vi "configure.vi"(8 "error in (no error)":errorcluster, 11 "PackedLibrary in":refnum<class "PackedLibrary.lvclass">) -> (0 "error out":errorcluster, 3 "PackedLibrary out":refnum<class "PackedLibrary.lvclass">)   [LabVIEW 2024, in "PackedLibrary.lvclass"]
uses:
  PackedLibrary.lvclass
  PackedLibrary.lvclass/PackedLibrary.ctl
  <vilib>/AppBuilder/AB_API/PPL/NI_AB_API_PPL.lvclass
  parent/Builder.lvclass
  D:/_repos/sandbox/github_p/labview-tools/cicd_tools/src/builders/parent/Builder.lvclass
  D:/_repos/sandbox/github_p/labview-tools/cicd_tools/src/builders/packed_library/PackedLibrary.lvclass
  C:/Program Files/National Instruments/LabVIEW 2024/vi.lib/AppBuilder/AB_API/Targetfile/NI_AB_API_Targetfile.lvclass
  C:/Program Files/National Instruments/LabVIEW 2024/vi.lib/AppBuilder/AB_API/Build/NI_AB_API_Build.lvclass
  C:/Program Files/National Instruments/LabVIEW 2024/vi.lib/AppBuilder/AB_API/PPL/NI_AB_API_PPL.lvclass
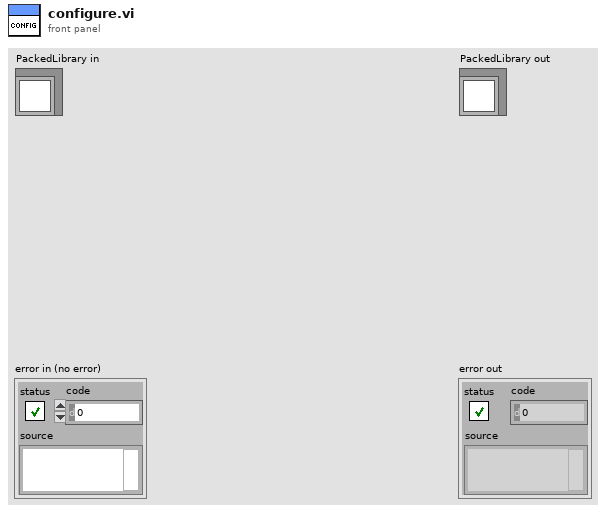
[diagram p1: front panel]
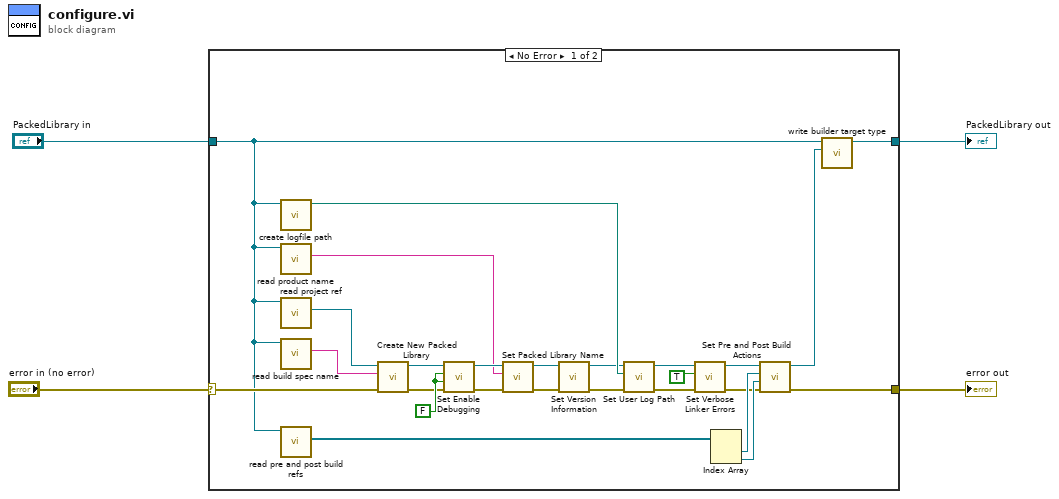
[diagram p0: block diagram]
diagram:
  n1 = case shown="No Error" "error in (no error)" {
    selector: "error in (no error)" -> [w12 w32]
    tunnel: [w13 w32] -> w4
    tunnel: [w7 w31] -> w2
    tunnel: "PackedLibrary in" -> [w6 w31]
    frame No Error {
      w20 = FALSE ("Enable debugging (false)")
      n2 = call "create logfile path.vi"("PackedLibrary in"=w6) -> ("logfile path"=w28:path)  [unwired: 10 in]
      n3 = call "read product name.vi"("Builders in"=w6) -> ("product name"=w5:string)  [unwired: 10 in]
      n4 = call "read project ref.vi"("Builders in"=w6) -> ("project ref"=w10:refnum<vi>)  [unwired: 10 in]
      n5 = call "read build spec name.vi"("Builders in"=w6) -> ("build spec name"=w11:string)  [unwired: 10 in]
      n6 = call "read pre and post build refs .vi"("Builders in"=w6) -> ("pre and post build refs"=w8:refnum<vi>[])  [unwired: 10 in]
      n7 = call <vilib>:"Create New Packed Library.vi"("error in (no error)"=w12, "Build specification name"=w11, "Project Refnum"=w10) -> ("error out"=w17:errorcluster, "PPL out"=w19:refnum<class "NI_AB_API_PPL.lvclass">)  [unwired: 7 in]
      n8 = call-dynamic "Set Enable Debugging.vi"("error in (no error)"=w17, "Wait for debugger on launch (false)"=w20, "Enable debugging (false)"=w20, "PPL in"=w19) -> ("error out"=w18:errorcluster, "PPL out"=w21:refnum<class "NI_AB_API_PPL.lvclass">)  [unwired: 6 in]
      n9 = call-dynamic "Set Packed Library Name.vi"("error in (no error)"=w18, "Packed library name"=w5, "PPL in"=w21) -> ("error out"=w23:errorcluster, "PPL out"=w22:refnum<class "NI_AB_API_PPL.lvclass">)  [unwired: 7 in]
      n10 = call-dynamic "Set Version Information.vi"("error in (no error)"=w23, "PPL in"=w22) -> ("error out"=w25:errorcluster, "PPL out"=w24:refnum<class "NI_AB_API_PPL.lvclass">)  [unwired: 8 in]
      n11 = call-dynamic "Set User Log Path.vi"("error in (no error)"=w25, "user log path"=w28, "NI_AB_API_PPL in"=w24) -> ("error out"=w26:errorcluster, "NI_AB_API_PPL out"=w27:refnum<class "NI_AB_API_PPL.lvclass">)  [unwired: 7 in]
      n12 = call-dynamic "Set Verbose Linker Errors.vi"("error in (no error)"=w26, "Verbose Linker Errors? (true)"=TRUE, "PPL in"=w27) -> ("error out"=w15:errorcluster, "PPL out"=w16:refnum<class "NI_AB_API_PPL.lvclass">)  [unwired: 7 in]
      n13 = Index Array(array=w8) -> (element #1=w29:refnum<vi>, element #2=w30:refnum<vi>)  [unwired: 2 in]
      n14 = call-dynamic "Set Pre and Post Build Actions.vi"("error in (no error)"=w15, "Post Build Action VI"=w30, "Pre Build Action VI"=w29, "Build in"=w16) -> ("error out"=w13:errorcluster, "Build out"=w9:refnum<class "NI_AB_API_PPL.lvclass">)  [unwired: 6 in]
      n15 = call "write builder target type.vi"("builder target type"=w9, "Builder in"=w6) -> ("Builder out"=w7:refnum<class "PackedLibrary.lvclass">)  [unwired: 9 in]
    }
    frame Error {
    }
  }
  "error out" <- w4
  "PackedLibrary out" <- w2
